vi "setInitTime.vi"(8 "error in (no error)":errorcluster, 11 "Model in":refnum<class "Model.lvclass">) -> (0 "error out":errorcluster, 3 "Model out":refnum<class "Model.lvclass">)   [LabVIEW 2016, in "Model.lvclass"]
uses:
  Model.lvclass
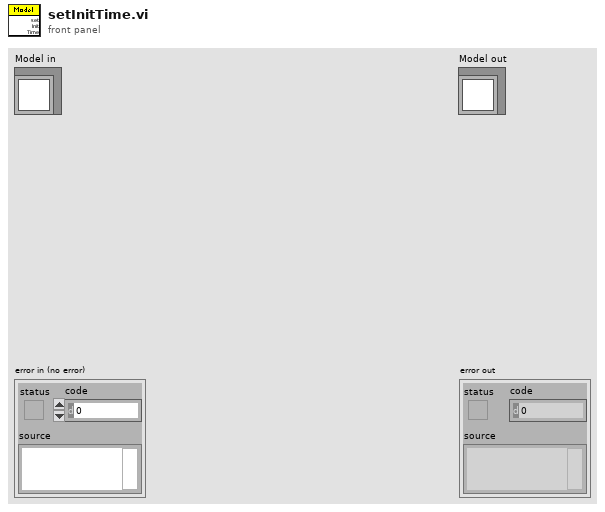
[diagram p1: front panel]
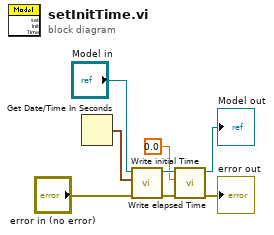
[diagram p0: block diagram]
diagram:
  n1 = Get Date/Time In Seconds() -> (seconds since 1Jan1904=w8:timestamp)
  n2 = call-dynamic "Write initial Time.vi"("error in (no error)"="error in (no error)", "initial Time"=w8, "Model in"="Model in") -> ("error out"=w4:errorcluster, "Model out"=w5:refnum<class "Model.lvclass">)  [unwired: 7 in]
  n3 = call-dynamic "Write elapsed Time.vi"("error in (no error)"=w4, "elapsed Time"=0.0, "Model in"=w5) -> ("error out"=→"error out":errorcluster, "Model out"=→"Model out":refnum<class "Model.lvclass">)  [unwired: 7 in]
